vi "Read from Data Source.vi"(8 "error in (no error)":errorcluster, 11 "INI in":refnum<class "Projects-INI.lvclass">) -> (0 "error out":errorcluster, 3 "INI out":refnum<class "Projects-INI.lvclass">)   [LabVIEW 2020, in "Projects-INI.lvclass"]
doc: "Reads data from the source location that the data is in. When this is called the map data for any projects that are already in the class data should be overwritten or added if they are not present. Becasue this is using the LabVIEW INI file read VIs, this will also automatically create the file if it does not already exist.\n\n03/2025 Erich Schlieper"
uses:
  Projects-INI.lvclass
  Projects-INI.lvclass/Projects-INI.ctl
  <vilib>/Utility/config.llb/NI_LVConfig.lvlib
  <vilib>/Utility/config.llb/Read Key (String).vi
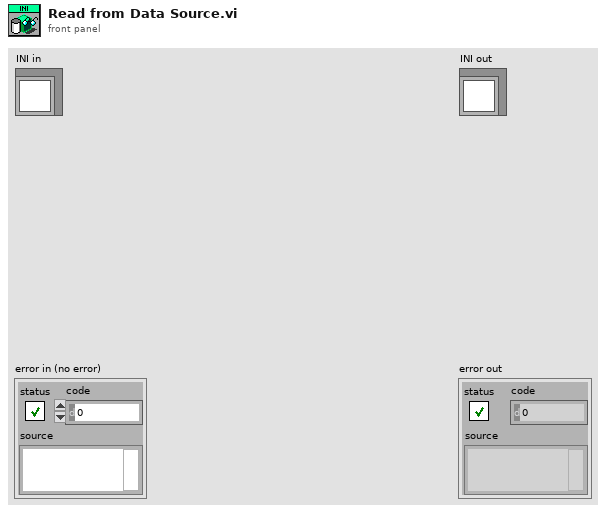
[diagram p1: front panel]
types:
  T1 = typedef "NI_LVConfig.lvlib/Config Data RefNum.ctl" = refnum<k1>
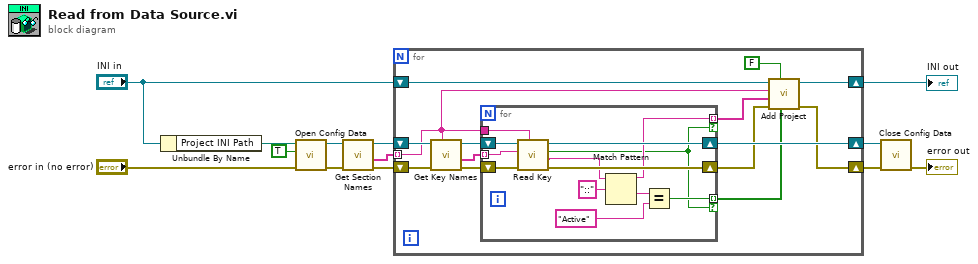
[diagram p0: block diagram]
diagram:
  n1 = Unbundle By Name("INI in") -> ("Project INI Path"=w1:path)
  n2 = call <vilib>:"Open Config Data.vi"("error in (no error)"="error in (no error)", "create file if necessary (T)"=TRUE, "configuration file path"=w1) -> ("error out"=w10:errorcluster, "refnum"=w11:T1)  [unwired: 6 in, 1 out]
  n3 = call <vilib>:"Get Section Names.vi"("error in (no error)"=w10, "refnum"=w11) -> ("error out"=w9:errorcluster, "section names"=w7:string[], "refnum out"=w8:T1)  [unwired: 7 in]
  n4 = for {
    shift-right: [w22] -> w3
    shift-left: w8 -> [w27]
    shift-right: [w20] -> w5
    shift-left: w9 -> [w26]
    tunnel: w7 -> [w17] mode=indexing
    shift-right: [w16] -> w6
    shift-left: "INI in" -> [w19]
    n5 = call <vilib>:"Get Key Names.vi"("section"=w17, "error in (no error)"=w26, "refnum"=w27) -> ("error out"=w24:errorcluster, "key names"=w23:string[], "refnum out"=w25:T1)  [unwired: 5 in, 1 out]
    n6 = for {
      shift-right: [w35] -> w22
      shift-left: w25 -> [w40]
      shift-right: [w36] -> w21
      shift-left: w24 -> [w39]
      tunnel: w23 -> [w38] mode=indexing
      tunnel: w17 -> [w37]
      tunnel: [w32] -> w18 mode=indexing if=w28
      tunnel: [w29] -> w14 mode=indexing if=w28
      n7 = call-poly <vilib>:"Read Key.vi"("section"=w37, "error in (no error)"=w39, "key"=w38, "refnum"=w40) -> ("error out"=w36:errorcluster, "value"=w33:string, "found?"=w28:bool, "refnum out"=w35:T1)  [unwired: 4 in]
      n8 = Match Pattern(string=w33, regular expression="::") -> (before substring=w32:string, after substring=w31:string)  [unwired: 1 in, 2 out]
      n9 = Equal?(x=w31, y="Active" ("regular expression")) -> (x = y?=w29:bool)
    }
    n10 = call-dynamic "Add Project.vi"("Tasks Active?"=w14, "Add Default Tasks (T)"=FALSE, "error in (no error)"=w21, "Tasks"=w18, "Project Name"=w17, "Projects in"=w19) -> ("error out"=w20:errorcluster, "Projects out"=w16:refnum<class "Projects-INI.lvclass">)  [unwired: 4 in]
  }
  "INI out" <- w6
  n11 = call <vilib>:"Close Config Data.vi"("error in (no error)"=w5, "refnum"=w3) -> ("error out"=→"error out":errorcluster)  [unwired: 8 in, 1 out]
